vi "Global 1.vi"() -> ()   [LabVIEW 2021]
panel:
  out "state":bool
  out "Robotic Hand Address":string="192.168.4.93"
  out "Glove output RT":dbl[](array[numeric])
  out "glove error out":errorcluster
  out "glove connection ID":refnum<k5>
  out "Glove Status":bool
  out "Robotic Hand Status":bool
  out "robotic hand error out":errorcluster
  out "robotic hand connection ID":refnum<k5>
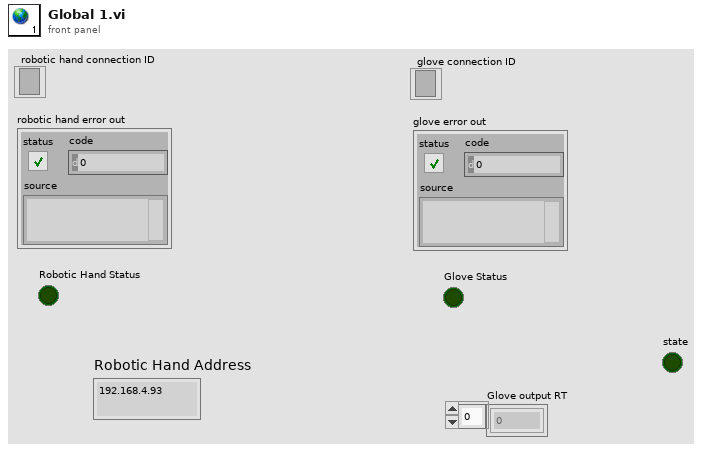
[diagram p1: front panel]
diagram:
